vi "1DCamera.vi"(9 "Angle3":bool, 10 "Angle2":bool, 11 "Angle1":bool) -> ()   [LabVIEW 2015]
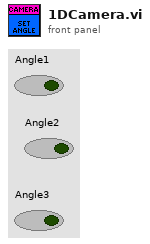
[diagram p1: front panel]
types:
  T1 = typedef "WPI_ServoDeviceRef.ctl" = cluster{"DeviceStatus":errorcluster, "PWM Channel":T2, "DeadBand":T3}
  T2 = typedef "FPGA_DIOPWMChannel.ctl" = enum8{"PWM 0", "PWM 1", "PWM 2", "PWM 3", "PWM 4", "PWM 5", "PWM 6", "PWM 7", "PWM 8", "PWM 9", "PWM MXP 0", "PWM MXP 1", "PWM MXP 2", "PWM MXP 3", "PWM MXP 4", "PWM MXP 5", "PWM MXP 6", "PWM MXP 7", "PWM MXP 8", "PWM MXP 9", "Invalid"}
  T3 = typedef "WPI_PWMDeadband.ctl" = cluster{"Name":string, "maxPositivePwm":i32, "minPositivePwm":i32, "centerPwm":i32, "maxNegativePwm":i32, "minNegativePwm":i32, "angularRange":u16}
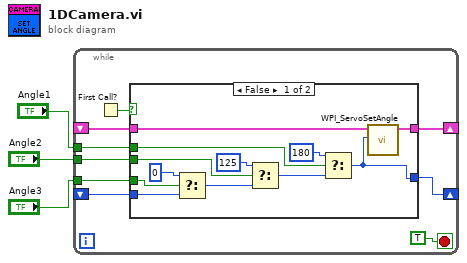
[diagram p0: block diagram]
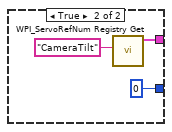
[diagram p2: hidden frame]
diagram:
  n1 = while {
    shift-right: [w10] -> _
    shift-left: _ -> [w6]
    shift-right: [w9] -> _
    shift-left: _ -> [w8]
    tunnel: "Angle3" -> [w7]
    tunnel: "Angle1" -> [w5]
    tunnel: "Angle2" -> [w4]
    stop <- TRUE stop-if-true
    n2 = First Call?() -> (First Call?: T/F=w11:bool)
    n3 = case shown="False" w11 {
      tunnel: [w17 w26] -> w10
      tunnel: [w20 0 ("t")] -> w9
      tunnel: w8 -> [w21 _]
      tunnel: w7 -> [w19 _]
      tunnel: w6 -> [w18 _]
      tunnel: w5 -> [w14 _]
      tunnel: w4 -> [w13 _]
      frame False {
        n4 = Select(t=0, s=w19, f=w21) -> (s? t:f=w24:i32)
        n5 = Select(t=125, s=w13, f=w24) -> (s? t:f=w23:i32)
        n6 = Select(t=180, s=w14, f=w23) -> (s? t:f=w20:i32)
        n7 = call <vilib>:"WPI_ServoSetAngle.vi"("Angle"=w20, "ServoDeviceRef"=w18) -> ("ServoDeviceRef"=w17:T1)  [unwired: 8 in, 1 out]
      }
      frame True {
        n8 = call <vilib>:"WPI_ServoRefNum Registry Get.vi"("refnum name"="CameraTilt") -> ("ServoDeviceRef"=w26:T1)  [unwired: 9 in, 1 out]
      }
    }
  }
